vi "Data Class_2D Str.vi"(5 "삭제?(F)":bool, 7 "인덱스":i32, 9 "대체 문자열":string, 10 "DATA 입력":string[][](array[string]), 11 "검색 문자열":string) -> (0 "제외 DATA 출력":string[][](array[string]), 1 "열크기":i32, 2 "행크기":i32, 3 "DATA 출력":string[][](array[string]), 4 "같음?":bool caption="<-같음?->")   [LabVIEW 2020]
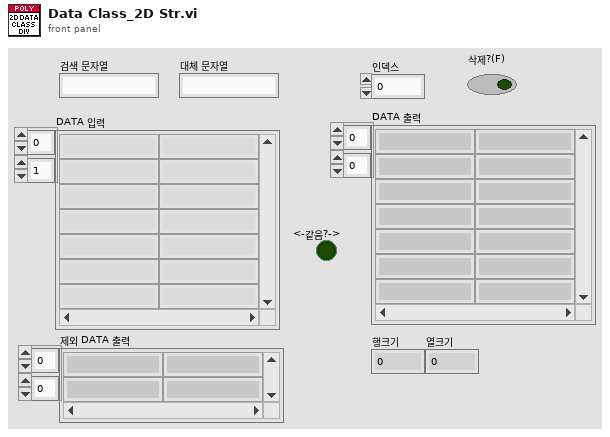
[diagram p1: front panel]
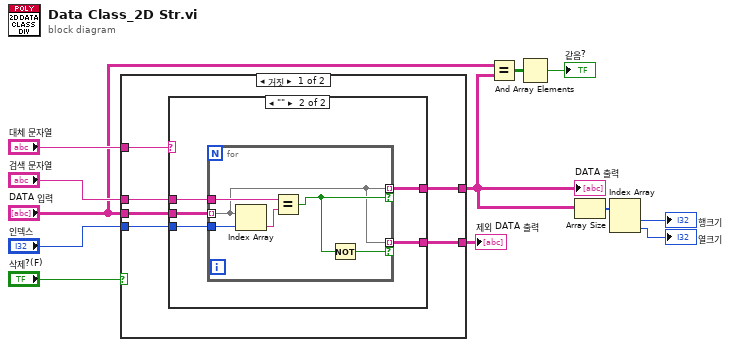
[diagram p0: block diagram]
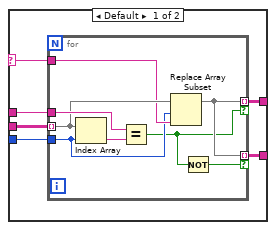
[diagram p2: hidden frame]
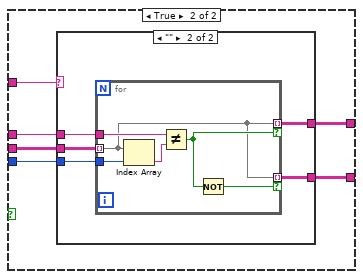
[diagram p3: hidden frame]
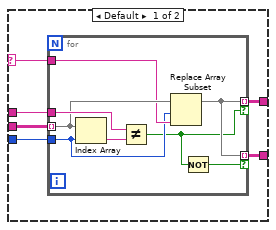
[diagram p4: hidden frame]
diagram:
  n1 = case shown="거짓" "삭제?(F)" {
    tunnel: "인덱스" -> [w18 w49]
    tunnel: [w17 w48] -> w3
    tunnel: "검색 문자열" -> [w16 w47]
    tunnel: "DATA 입력" -> [w15 w46]
    tunnel: "대체 문자열" -> [w14 w45]
    tunnel: [w13 w44] -> w5
    frame False {
      n2 = case shown="\"\"" w14 {
        selector: w14 -> [w20 _]
        tunnel: w18 -> [w24 w37]
        tunnel: [w23 w36] -> w17
        tunnel: w16 -> [w22 w35]
        tunnel: w15 -> [w21 w34]
        tunnel: [w19 w33] -> w13
        frame Default {
          n3 = for {
            tunnel: w21 -> [w30] mode=indexing
            tunnel: w22 -> [w32]
            tunnel: [w27] -> w23 mode=indexing if=w25
            tunnel: w24 -> [w28]
            tunnel: w20 -> [w29]
            tunnel: [w27] -> w19 mode=indexing if=w26
            n4 = Index Array(array=w30, index=w28) -> (element=w31:string)
            n5 = Equal?(x=w32, y=w31) -> (x = y?=w25:bool)
            n6 = Replace Array Subset(array=w30, new element=w29, index=w28) -> (w27:string[])
            n7 = Not(x=w25) -> (.not. x?=w26:bool)
          }
        }
        frame "" {
          n8 = for {
            tunnel: w34 -> [w39] mode=indexing
            tunnel: w35 -> [w43]
            tunnel: [w39] -> w36 mode=indexing if=w40
            tunnel: w37 -> [w41]
            tunnel: [w39] -> w33 mode=indexing if=w38
            n9 = Index Array(array=w39, index=w41) -> (element=w42:string)
            n10 = Equal?(x=w43, y=w42) -> (x = y?=w40:bool)
            n11 = Not(x=w40) -> (.not. x?=w38:bool)
          }
        }
      }
    }
    frame True {
      n12 = case shown="\"\"" w45 {
        selector: w45 -> [w51 _]
        tunnel: w49 -> [w55 w68]
        tunnel: [w54 w67] -> w48
        tunnel: w47 -> [w53 w66]
        tunnel: w46 -> [w52 w65]
        tunnel: [w50 w64] -> w44
        frame Default {
          n13 = for {
            tunnel: w52 -> [w61] mode=indexing
            tunnel: w53 -> [w63]
            tunnel: [w58] -> w54 mode=indexing if=w56
            tunnel: w55 -> [w59]
            tunnel: w51 -> [w60]
            tunnel: [w58] -> w50 mode=indexing if=w57
            n14 = Index Array(array=w61, index=w59) -> (element=w62:string)
            n15 = Not Equal?(x=w63, y=w62) -> (x != y?=w56:bool)
            n16 = Replace Array Subset(array=w61, new element=w60, index=w59) -> (w58:string[])
            n17 = Not(x=w56) -> (.not. x?=w57:bool)
          }
        }
        frame "" {
          n18 = for {
            tunnel: w65 -> [w70] mode=indexing
            tunnel: w66 -> [w74]
            tunnel: [w70] -> w67 mode=indexing if=w71
            tunnel: w68 -> [w72]
            tunnel: [w70] -> w64 mode=indexing if=w69
            n19 = Index Array(array=w70, index=w72) -> (element=w73:string)
            n20 = Not Equal?(x=w74, y=w73) -> (x != y?=w71:bool)
            n21 = Not(x=w71) -> (.not. x?=w69:bool)
          }
        }
      }
    }
  }
  "DATA 출력" <- w3
  "제외 DATA 출력" <- w5
  n22 = Equal?(x="DATA 입력", y=w3) -> (x = y?=w2:bool[][])
  n23 = And Array Elements(Boolean array=w2) -> (logical AND=→"같음?":bool)
  n24 = Array Size(array=w3) -> (size(s)=w8:i32[])
  n25 = Index Array(array=w8) -> (element #1=→"행크기":i32, element #2=→"열크기":i32)  [unwired: 2 in]
